vi "DatabaseHand_FlushQvar.vi"(8 "error in (no error)":errorcluster, 10 "name":string, 11 "Database RefNum In":T1) -> (0 "error out":errorcluster, 3 "Database RefNum out":T1)   [LabVIEW 2016]
doc: "This VI finds the RefNum of an existing object with the input Name or creates a new object if the Name is not found or Name is unwired or an empty string.\nCopyright 2001 VI Engineering, Inc."
uses:
  private/vis/DatabaseHand_RefNum.ctl
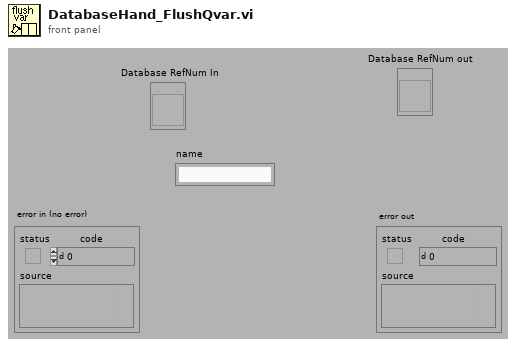
[diagram p1: front panel]
types:
  T1 = typedef "DatabaseHand_RefNum.ctl" = refnum<vi>
  T2 = typedef "DatabaseHand_Element.ctl" = cluster{"name":string, "Database":T3[]}
  T3 = typedef "DatabaseHan_DatabaseElement.ctl" = cluster{"name":string, "value":string, "type":string, "unit":string, "permissions":string, "enqueued":bool, "group":string}
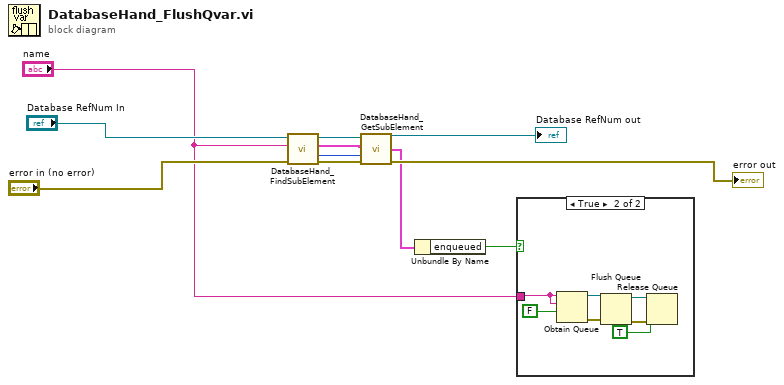
[diagram p0: block diagram]
diagram:
  n1 = call "DatabaseHand_FindSubElement.vi"("error in (no error)"="error in (no error)", "name"="name", "Database RefNum in"="Database RefNum In") -> ("error out"=w9:errorcluster, "index"=w8:i32, "Database"=w10:T2, "Database RefNum out"=w11:T1)  [unwired: 5 out]
  n2 = call "DatabaseHand_GetSubElement.vi"("Database RefNum in"=w11, "Object Data In"=w10, "Index"=w8, "error in (no error)"=w9) -> ("Database RefNum out"=→"Database RefNum out":T1, "Element found"=w3:T3, "error out"=→"error out":errorcluster)  [unwired: 1 in, 8 out]
  n3 = Unbundle By Name(w3) -> ("enqueued"=w2:bool)
  n4 = case shown="True" w2 {
    tunnel: "name" -> [_ w17]
    frame False {
    }
    frame True {
      n5 = Obtain Queue(name (unnamed)=w17, element data type=w17, create if not found? (T)=FALSE) -> (queue out=w16:refnum<queue>, error out=w15:errorcluster)  [unwired: 2 in, 1 out]
      n6 = Flush Queue(queue=w16, error in (no error)=w15) -> (queue out=w14:refnum<queue>, error out=w13:errorcluster)  [unwired: 1 out]
      n7 = Release Queue(queue=w14, force destroy? (F)=TRUE, error in (no error)=w13) -> ()  [unwired: 3 out]
    }
  }
